vi "JSON ParserDTCConfig.vi"(8 "Error In":errorcluster, 9 "NumElements":i32=24, 10 "jsonin":string, 11 "Sequence Context In":refnum<k7>) -> (0 "error out":errorcluster)   [LabVIEW 2017]
uses:
  <vilib>/addons/TestStand/_TSUtility.llb/TestStand - Set Property Value (Number).vi
  <vilib>/addons/TestStand/_TSUtility.llb/TestStand - Set Property Value (String).vi
  <vilib>/addons/TestStand/_TSUtility.llb/TestStand - Set Property Value (Boolean).vi
  <vilib>/addons/TestStand/_TSUtility.llb/TestStand - Set Property Value (Boolean Array).vi
panel:
  out "Array":string[](array[string])
  out "ParameterType":string[](array[string])
  out "error out 2":errorcluster
  out "result string":string
  out "Parameter Name":string[](array[string])
  out "Value":string[](array[string])
  out "DataTrype":string[](array[string])
  out "Parameter Set":string
  out "output array":string[][](array[string])
  out "Param Values":string[](array[string])
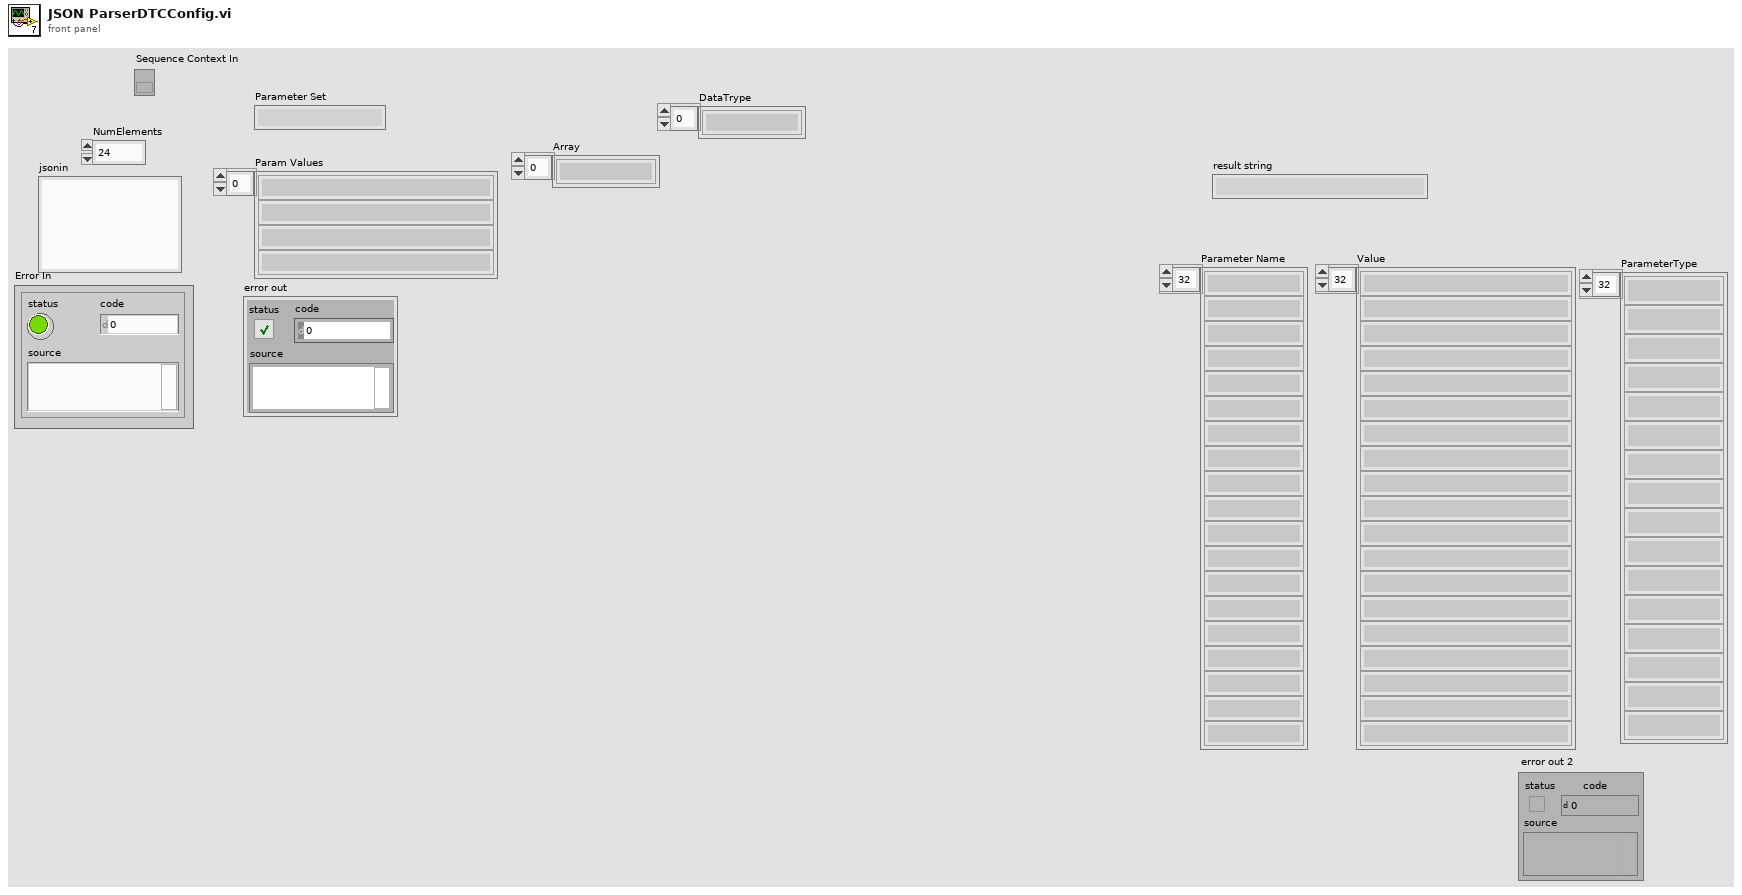
[diagram p1: front panel]
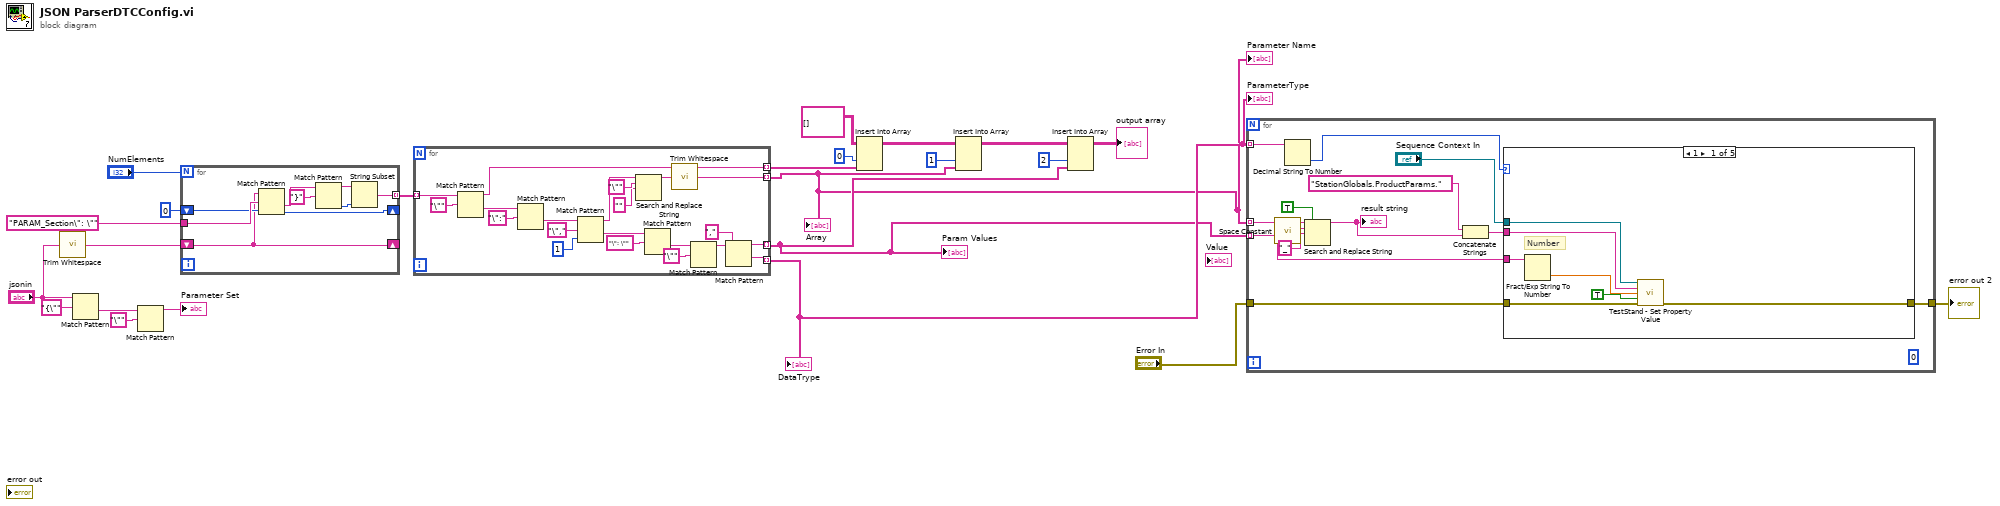
[diagram p0: block diagram]
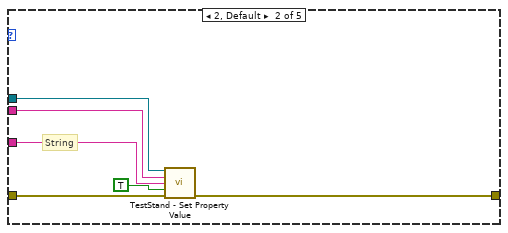
[diagram p2: hidden frame]
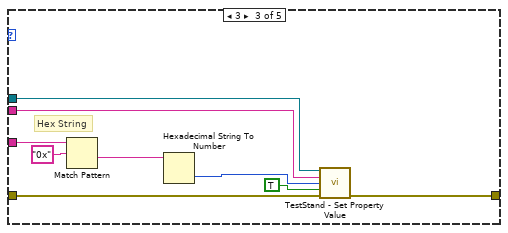
[diagram p3: hidden frame]
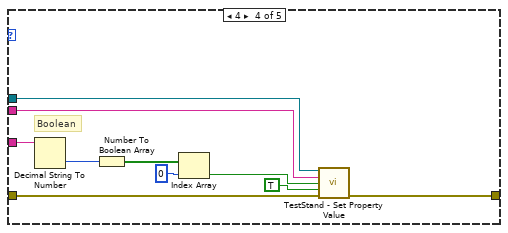
[diagram p4: hidden frame]
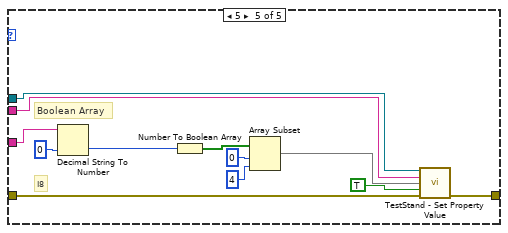
[diagram p5: hidden frame]
diagram:
  n1 = call <vilib>:"Trim Whitespace.vi"("string"="jsonin") -> ("trimmed string"=w20:string)  [unwired: 1 in]
  n2 = Match Pattern(string="jsonin", regular expression="{\"") -> (after substring=w9:string)  [unwired: 1 in, 3 out]
  n3 = Match Pattern(string=w9, regular expression="\"") -> (before substring=→"Parameter Set":string)  [unwired: 1 in, 3 out]
  n4 = for {
    N: "NumElements" -> [_]
    tunnel: "PARAM_Section\": \"" ("regular expression") -> [w32]
    shift-right: [w25] -> _
    shift-left: 0 -> [w26]
    tunnel: [w28] -> w21 mode=indexing
    shift-right: [w24] -> _
    shift-left: w20 -> [w24]
    n5 = Match Pattern(string=w24, regular expression=w32, offset (0)=w26) -> (after substring=w31:string, offset past match=w25:i32)  [unwired: 2 out]
    n6 = Match Pattern(string=w31, regular expression="}") -> (before substring=w29:string, offset past match=w27:i32)  [unwired: 1 in, 2 out]
    n7 = String Subset(string=w29, length (rest)=w27) -> (substring=w28:string)  [unwired: 1 in]
  }
  n8 = for {
    tunnel: w21 -> [w40] mode=indexing
    tunnel: [w35] -> w2 mode=indexing
    tunnel: [w38] -> w17 mode=indexing
    tunnel: [w37] -> w1 mode=indexing
    tunnel: [w34] -> w3 mode=indexing
    n9 = Match Pattern(string=w40, regular expression="\"") -> (before substring=w38:string, after substring=w52:string)  [unwired: 1 in, 2 out]
    n10 = Match Pattern(string=w52, regular expression="\":") -> (after substring=w50:string)  [unwired: 1 in, 3 out]
    n11 = Match Pattern(string=w50, regular expression="\",", offset (0)=1) -> (before substring=w47:string, after substring=w43:string)  [unwired: 2 out]
    n12 = Search and Replace String(input string=w47, search string="\"", replace string="" ("replace string (\"\")")) -> (result string=w44:string)  [unwired: 5 in, 3 out]
    n13 = Match Pattern(string=w43, regular expression="\": \"") -> (after substring=w39:string)  [unwired: 1 in, 3 out]
    n14 = call <vilib>:"Trim Whitespace.vi"("string"=w44) -> ("trimmed string"=w37:string)  [unwired: 1 in]
    n15 = Match Pattern(string=w39, regular expression="\"") -> (before substring=w36:string)  [unwired: 1 in, 3 out]
    n16 = Match Pattern(string=w36, regular expression=",") -> (before substring=w35:string, after substring=w34:string)  [unwired: 1 in, 2 out]
  }
  "Param Values" <- w2
  "DataTrype" <- w3
  "Parameter Name" <- w1
  "ParameterType" <- w3
  "Array" <- w1
  n17 = Insert Into Array(array=string[][] [], index (col)=0 ("disabled index (col)"), new element=w17) -> (w15:string[][])  [unwired: 1 in]
  n18 = Insert Into Array(array=w15, index (col)=1 ("disabled index (col)"), new element=w1) -> (w13:string[][])  [unwired: 1 in]
  n19 = Insert Into Array(array=w13, index (col)=2 ("disabled index (col)"), new element=w2) -> (→"output array":string[][])  [unwired: 1 in]
  n20 = for {
    tunnel: w2 -> [w61] mode=indexing
    tunnel: w3 -> [w59] mode=indexing
    tunnel: [w55] -> w5
    tunnel: "Error In" -> [w56]
    tunnel: w1 -> [w60] mode=indexing
    (unwired) 0 ("y")
    n21 = call <vilib>:"Space Constant.vi"() -> ("String"=w65:string)
    n22 = Decimal String To Number(string=w59) -> (number=w54:i32)  [unwired: 2 in, 1 out]
    n23 = Search and Replace String(replace all?=TRUE ("replace all? (F)"), input string=w60, search string=w65, replace string="_" ("replace string (\"\")")) -> (result string=w63:string)  [unwired: 1 in, 6 out]
    "result string" <- w63
    n24 = Concatenate Strings("StationGlobals.ProductParams." ("Lookup String"), w63) -> (w57:string)
    n25 = case shown="1" w54 {
      tunnel: w61 -> [w73 w74 w82 w93 w105]
      tunnel: "Sequence Context In" -> [w72 w79 w88 w98 w110]
      tunnel: w57 -> [w71 w78 w87 w97 w109]
      tunnel: w56 -> [w69 w76 w85 w95 w107]
      tunnel: [w68 w75 w84 w94 w106] -> w55
      frame 1 {
        # "Number"
        n26 = Fract/Exp String To Number(string=w73) -> (number=w67:dbl)  [unwired: 4 out]
        n27 = call-poly <vilib>:"TestStand - Set Property Value.vi"("Sequence Context In"=w72, "Lookup String"=w71, "New Value"=w67, "Insert If Missing"=TRUE, "error in (no error)"=w69) -> ("error out"=w68:errorcluster)  [unwired: 10 out]
      }
      frame 2, Default {
        # "String"
        n28 = call-poly <vilib>:"TestStand - Set Property Value.vi"("Sequence Context In"=w79, "Lookup String"=w78, "New Value"=w74, "Insert If Missing"=TRUE, "error in (no error)"=w76) -> ("error out"=w75:errorcluster)  [unwired: 10 out]
      }
      frame 3 {
        # "Hex String"
        n29 = Match Pattern(string=w82, regular expression="0x") -> (after substring=w80:string)  [unwired: 1 in, 3 out]
        n30 = Hexadecimal String To Number(string=w80) -> (number=w83:u32)  [unwired: 2 in, 1 out]
        n31 = call-poly <vilib>:"TestStand - Set Property Value.vi"("Sequence Context In"=w88, "Lookup String"=w87, "New Value"=w83, "Insert If Missing"=TRUE, "error in (no error)"=w85) -> ("error out"=w84:errorcluster)  [unwired: 10 out]
      }
      frame 4 {
        # "Boolean"
        n32 = Decimal String To Number(string=w93) -> (number=w89:i32)  [unwired: 2 in, 1 out]
        n33 = Number To Boolean Array(number=w89) -> (Boolean array=w92:bool[])
        n34 = Index Array(array=w92, index=0) -> (element=w90:bool)
        n35 = call-poly <vilib>:"TestStand - Set Property Value.vi"("Sequence Context In"=w98, "Lookup String"=w97, "New Value"=w90, "Insert If Missing"=TRUE, "error in (no error)"=w95) -> ("error out"=w94:errorcluster)  [unwired: 10 out]
      }
      frame 5 {
        # "I8"
        # "Boolean Array"
        n36 = Decimal String To Number(string=w105, default (0L)=i8 0 ("default (0 I32)")) -> (number=w99:i8)  [unwired: 1 in, 1 out]
        n37 = Number To Boolean Array(number=w99) -> (Boolean array=w103:bool[])
        n38 = Array Subset(array=w103, index=0, length=4 ("index")) -> (w100:bool[])
        n39 = call-poly <vilib>:"TestStand - Set Property Value.vi"("Sequence Context In"=w110, "Lookup String"=w109, "New Value"=w100, "Insert If Missing"=TRUE, "error in (no error)"=w107) -> ("error out"=w106:errorcluster)  [unwired: 10 out]
      }
    }
  }
  "error out 2" <- w5
